vi "SetStreamingFilter.vi"(8 "error in (no error)":errorcluster, 10 "IDs":T1, 11 "Ref in":T4) -> (0 "error out":errorcluster, 3 "Ref out":T4)   [LabVIEW 2019, in "Protection and Counter Host Automation API.lvlib"]
uses:
  Protection and Counter Host Automation API.lvlib
  Types/API Variables.ctl
  <vilib>/NI/STM/TCP/TCP Connection Info.ctl
  <vilib>/NI/STM/SubVIs/MetaDataElement.ctl
  SubModules/CAN-Streaming-Support/Addon/Addon Shared/Types/Filter Parameters.ctl
  SubModules/CAN-Streaming-Support/Addon/Addon Shared/Types/Direction Filter.ctl
  SubModules/CAN-Streaming-Support/Addon/Addon Shared/Types/Type Filter.ctl
  <vilib>/NI/NI VeriStand Addon Network Comm/Shared/NI VeriStand Addon Network Comm Shared.lvlib
  <vilib>/NI/STM/NI STM.lvlib
  SubModules/CAN-Streaming-Support/Addon/Addon Shared/CAN Stream Support Shared.lvlib
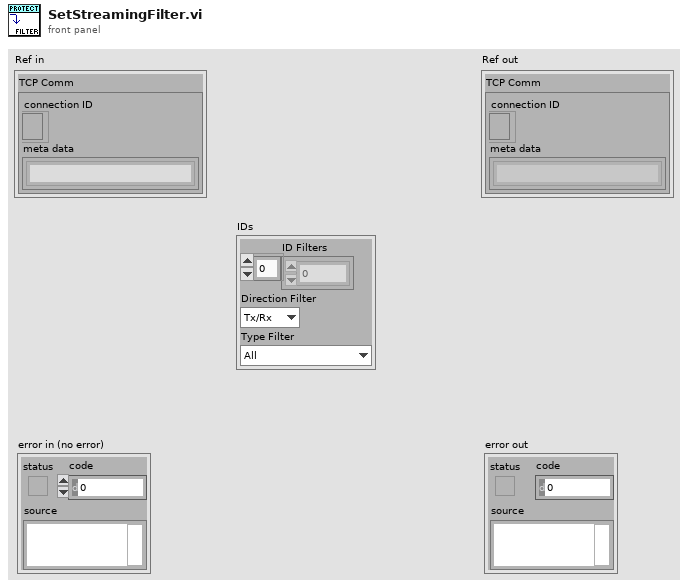
[diagram p1: front panel]
types:
  T1 = typedef "CAN Stream Support Shared.lvlib/Filter Parameters.ctl" = cluster{"ID Filters":u32[], "Direction Filter":T2, "Type Filter":T3}
  T2 = typedef "CAN Stream Support Shared.lvlib/Direction Filter.ctl" = enum16{"Tx/Rx", "Rx", "Tx"}
  T3 = typedef "CAN Stream Support Shared.lvlib/Type Filter.ctl" = enum16{"All", "CAN Data", "CAN Remote", "CAN Bus Error", "CAN 2.0 Data", "CAN FD Data", "CAN FD+BRS Data", "J1939 Data", "Delay", "Log Trigger", "Start Trigger"}
  T4 = typedef "Protection and Counter Host Automation API.lvlib/API Variables.ctl" = cluster{"TCP Comm":T5}
  T5 = typedef "NI STM.lvlib/TCP Connection Info.ctl" = cluster{"connection ID":refnum<k5>, "meta data":T6[]}
  T6 = typedef "NI STM.lvlib/MetaDataElement.ctl" = string
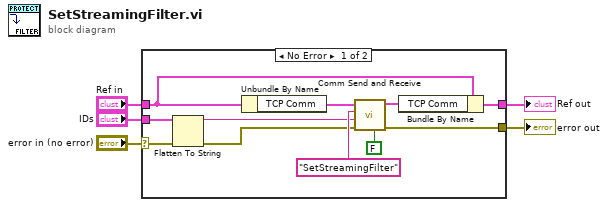
[diagram p0: block diagram]
diagram:
  n1 = case shown="No Error" "error in (no error)" {
    selector: "error in (no error)" -> [w9 w18]
    tunnel: "Ref in" -> [w12 w17]
    tunnel: [w10 w17] -> w4
    tunnel: [w16 w18] -> w3
    tunnel: "IDs" -> [w7 _]
    frame No Error {
      n2 = Flatten To String(anything=w7, error in (no error)=w9) -> (data string=w6:string, error out=w8:errorcluster)  [unwired: 2 in, 1 out]
      n3 = Unbundle By Name(w12) -> ("TCP Comm"=w13:T5)
      n4 = call <vilib>:"Comm Send and Receive.vi"("Resp Required?"=FALSE, "error in (no error)"=w8, "Data"=w6, "Name"="SetStreamingFilter", "connection info"=w13) -> ("error out"=w16:errorcluster, "connection info"=w11:T5)  [unwired: 3 in, 2 out]
      n5 = Bundle By Name(cluster=w12, "TCP Comm"=w11) -> (w10:T4)
    }
    frame Error {
    }
  }
  "Ref out" <- w4
  "error out" <- w3
